vi "ValidateScanInput.vi"(0 "Original Scan":refnum<class "Scan.lvclass">, 1 "New Scan":refnum<class "Scan.lvclass">, 2 "Galvo Array":refnum<class "Galvonometer.lvclass">[](array[class])=[refnum, refnum], 3 "Camera.lvclass":refnum<class "Camera.lvclass">) -> (4 "Current Scan Schematic":cluster{dbl[], dbl[]}[](graph)=[{[-5.0, 5.0, 5.0, -5.0, -5.0], [5.0, 5.0, -5.0, -5.0, 5.0]}, {[-12.5, 12.5, 12.5, -12.5, -12.5], [12.5, 12.5, -12.5, -12.5, 12.5]}], 5 "Max file size exceeded":bool, 6 "Output scan":refnum<class "Scan.lvclass">, 7 "Memory (GB)":dbl=0.36864, 8 "Time (s)":sgl=0.72, 9 "Max Voltage Exceeded":bool)   [LabVIEW 2017]
uses:
  classes/Scans/Scan.lvclass
  classes/HardwareObjects/Galvonometer/Galvonometer.lvclass
  classes/HardwareObjects/Camera/Camera.lvclass
  classes/HardwareObjects/Camera/Camera.lvclass/Camera.ctl
  classes/HardwareObjects/Galvonometer/Galvonometer.lvclass/Galvonometer.ctl
  classes/Scans/Scan.lvclass/Scan.ctl
  classes/Scans/Write Scan Pattern.vi
  classes/Scans/Write C scans.vi
  classes/Scans/Write B scans.vi
  classes/Scans/Write Repeat B scans.vi
  classes/Scans/Write Bidirectional.vi
  classes/Scans/Write A scans.vi
  classes/Scans/Write Scan Angle (degrees).vi
  classes/Scans/Write X FOV (degrees).vi
  classes/Scans/Write X offset (degrees).vi
  classes/Scans/Write Y FOV (degrees).vi
  classes/Scans/Write Y offset (degrees).vi
  classes/HardwareObjects/Camera/Read Bit Depth.vi
  classes/HardwareObjects/Camera/Read Camera Dimensions.vi
  classes/HardwareObjects/Camera/Read Max Frequency (kHz).vi
  classes/HardwareObjects/Galvonometer/Read Max Scan Angle (degrees).vi
  classes/HardwareObjects/Galvonometer/Read Output Scale Factor (V_degrees).vi
  classes/Scans/Read Scan Pattern.vi
  classes/Scans/Read B scans.vi
  classes/Scans/Read A scans.vi
  classes/Scans/Read Scan Angle (degrees).vi
  classes/Scans/Read X FOV (degrees).vi
  classes/Scans/Read X offset (degrees).vi
  classes/Scans/Read Y FOV (degrees).vi
  classes/Scans/Read Y offset (degrees).vi
  classes/Scans/Read Total A-scans per volume.vi
panel:
  in  "stop":bool
  in  "debug":bool
  in  "Y offset (degrees)":dbl
  in  "Y FOV (degrees)":dbl=10.0
  in  "X offset (degrees)":dbl
  in  "X FOV (degrees)":dbl=10.0
  in  "Scan Angle (degrees)":dbl
  in  "A scans":dbl=300.0
  in  "Bidirectional":bool
  in  "Repeat B scans":dbl=1.0
  in  "B scans":dbl=300.0
  in  "C scans":dbl=1.0
  in  "Scan Pattern":string="Rectangle"
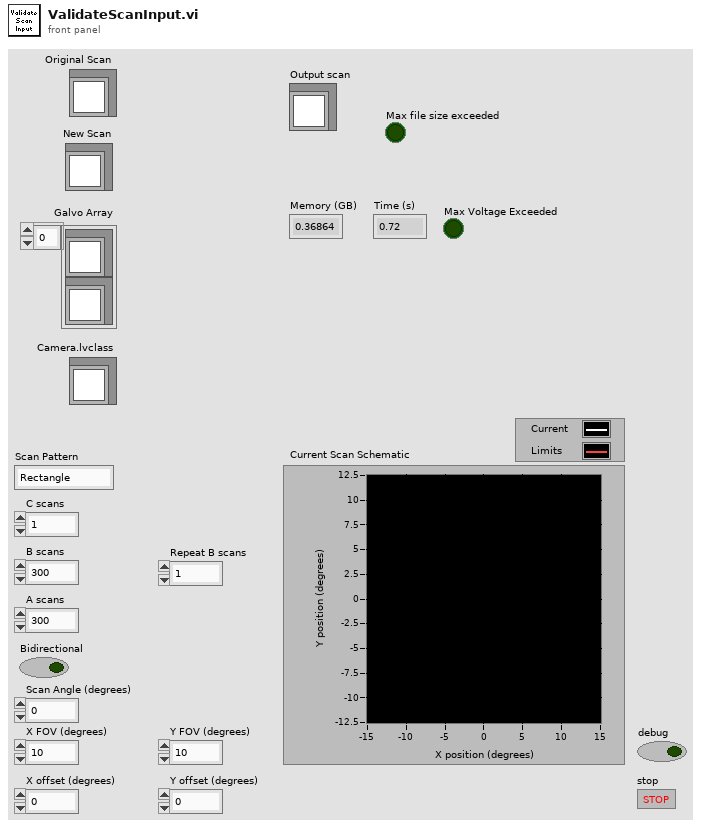
[diagram p1: front panel]
types:
  T1 = cluster{"X FOV (degrees)":dbl, "X offset (degrees)":dbl, "Y FOV (degrees)":dbl, "Y offset (degrees)":dbl}
  T2 = cluster{"X FOV (degrees)":dbl, "Y FOV (degrees)":dbl}
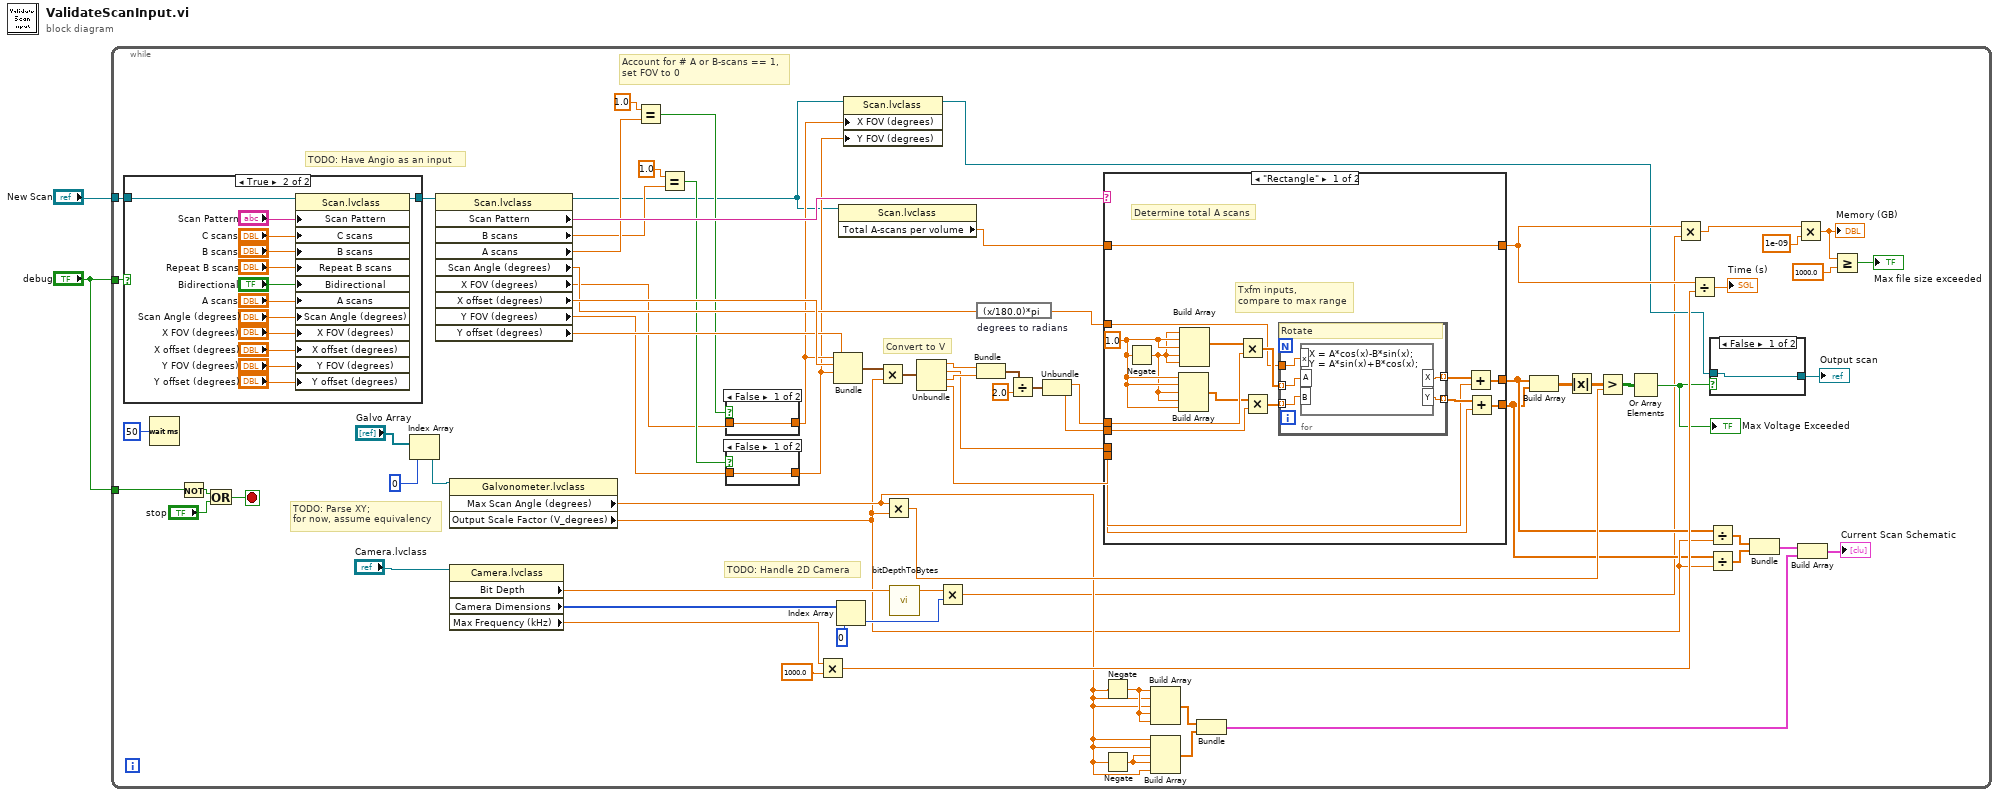
[diagram p0: block diagram]
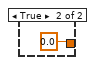
[diagram p2: hidden frame]
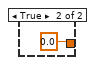
[diagram p3: hidden frame]
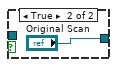
[diagram p5: hidden frame]
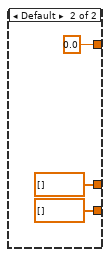
[diagram p6: hidden frame]
diagram:
  n1 = while {
    tunnel: "New Scan" -> [w33]
    tunnel: "debug" -> [w31]
    tunnel: "debug" -> [w29]
    stop <- w27 stop-if-true
    # "Account for # A or B-scans == 1,\nset FOV to 0"
    # "TODO: Have Angio as an input"
    # "TODO: Handle 2D Camera"
    # "Convert to V"
    # "TODO: Parse XY;\nfor now, assume equivalency"
    n2 = case shown="True" w31 {
      tunnel: w33 -> [w83 w85]
      tunnel: [w83 w84] -> w32
      frame False {
      }
      frame True {
        n3 = property class="Scan.lvclass"(reference=w85, "Scan Pattern"="Scan Pattern", "C scans"="C scans", "B scans"="B scans", "Repeat B scans"="Repeat B scans", "Bidirectional"="Bidirectional", "A scans"="A scans", "Scan Angle (degrees)"="Scan Angle (degrees)", "X FOV (degrees)"="X FOV (degrees)", "X offset (degrees)"="X offset (degrees)", "Y FOV (degrees)"="Y FOV (degrees)", "Y offset (degrees)"="Y offset (degrees)") -> (reference out=w84:refnum<class "Scan.lvclass">)  [unwired: 1 in, 1 out]
      }
    }
    n4 = Wait (ms)(milliseconds to wait=u32 50) -> ()  [unwired: 1 out]
    n5 = Not(x=w29) -> (.not. x?=w30:bool)
    n6 = Or(x=w30, y="stop") -> (x .or. y?=w27:bool)
    n7 = Index Array(array="Galvo Array", index=0) -> (element=w76:refnum<class "Galvonometer.lvclass">)
    n8 = property class="Scan.lvclass"(reference=w32) -> (reference out=w5:refnum<class "Scan.lvclass">, "Scan Pattern"=w74:string, "B scans"=w18:dbl, "A scans"=w20:dbl, "Scan Angle (degrees)"=w58:dbl, "X FOV (degrees)"=w15:dbl, "X offset (degrees)"=w73:dbl, "Y FOV (degrees)"=w14:dbl, "Y offset (degrees)"=w72:dbl)  [unwired: 1 in, 1 out]
    n9 = property class="Galvonometer.lvclass"(reference=w76) -> ("Max Scan Angle (degrees)"=w40:dbl, "Output Scale Factor (V_degrees)"=w39:dbl)  [unwired: 1 in, 2 out]
    n10 = property class="Camera.lvclass"(reference="Camera.lvclass") -> ("Bit Depth"=w68:dbl, "Camera Dimensions"=w70:u16[], "Max Frequency (kHz)"=w48:sgl)  [unwired: 1 in, 2 out]
    n11 = Equal?(x=1.0, y=w20) -> (x = y?=w17:bool)
    n12 = Equal?(x=1.0, y=w18) -> (x = y?=w16:bool)
    n13 = case shown="False" w17 {
      tunnel: w15 -> [w81 _]
      tunnel: [w81 0.0 ("X FOV (degrees)")] -> w13
      frame False {
      }
      frame True {
      }
    }
    n14 = case shown="False" w16 {
      tunnel: w14 -> [w79 _]
      tunnel: [w79 0.0 ("Y FOV (degrees)")] -> w12
      frame False {
      }
      frame True {
      }
    }
    n15 = Multiply(x=w48, y=1000.0) -> (x*y=w47:dbl)
    n16 = Bundle("X FOV (degrees)"=w13, "X offset (degrees)"=w73, "Y FOV (degrees)"=w12, "Y offset (degrees)"=w72) -> (w71:T1)  [unwired: 1 in]
    n17 = Index Array(array=w70, index=0) -> (element=w67:u16)
    n18 = property class="Scan.lvclass"(reference=w5) -> ("Total A-scans per volume"=w4:dbl)  [unwired: 1 in, 2 out]
    n19 = property class="Scan.lvclass"(reference=w5, "X FOV (degrees)"=w13, "Y FOV (degrees)"=w12) -> (reference out=w11:refnum<class "Scan.lvclass">)  [unwired: 1 in, 1 out]
    n20 = Multiply(x=w71, y=w39) -> (x*y=w66:T1)
    n21 = Multiply(x=w40, y=w39) -> (x*y=w53:dbl)
    n22 = call "bitDepthToBytes.vi"("bit depth"=w68) -> ("bytes"=w10:dbl)  [unwired: 9 in]
    n23 = Unbundle(w66) -> ("X FOV (degrees)"=w63:dbl, "X offset (degrees)"=w56:dbl, "Y FOV (degrees)"=w62:dbl, "Y offset (degrees)"=w55:dbl)
    n24 = Multiply(x=w10, y=w67) -> (x*y=w3:dbl)
    n25 = Bundle("X FOV (degrees)"=w63, "Y FOV (degrees)"=w62) -> (w64:T2)  [unwired: 1 in]
    n26 = expression code="(x/180.0)*pi" "degrees to radians"(w58) -> (w57:dbl)
    n27 = Divide(x=w64, y=2.0) -> (x/y=w61:T2)
    n28 = Unbundle(w61) -> ("X FOV (degrees)"=w60:dbl, "Y FOV (degrees)"=w59:dbl)
    n29 = Negate(x=w40) -> (-x=w41:dbl)
    n30 = Negate(x=w40) -> (-x=w43:dbl)
    n31 = case shown="\"Rectangle\"" w74 {
      tunnel: w60 -> [w113 _]
      tunnel: w59 -> [w112 _]
      tunnel: w57 -> [w109 _]
      tunnel: w56 -> [w106 _]
      tunnel: w55 -> [w105 _]
      tunnel: [w104 dbl[] []] -> w24
      tunnel: [w99 0.0] -> w46
      tunnel: [w103 dbl[] []] -> w23
      tunnel: w4 -> [w99 _]
      frame "Rectangle" {
        w102 = 1.0 ("element")
        # "Txfm inputs,\ncompare to max range"
        # "Determine total A scans"
        n32 = Negate(x=w102) -> (-x=w101:dbl)
        n33 = Build Array(w102, w102, w101, w101, w102) -> (w100:dbl[])
        n34 = Build Array(w101, w102, w102, w101, w101) -> (w114:dbl[])
        n35 = Multiply(x=w114, y=w113) -> (x*y=w111:dbl[])
        n36 = Multiply(x=w100, y=w112) -> (x*y=w110:dbl[])
        n37 = for {
          tunnel: w111 -> [w119] mode=indexing
          tunnel: w109 -> [w118]
          tunnel: [w117] -> w108 mode=indexing
          tunnel: w110 -> [w116] mode=indexing
          tunnel: [w115] -> w107 mode=indexing
          # "Rotate"
          n38 = formula code="X = A*cos(x)-B*sin(x);\nY = A*sin(x)+B*cos(x);"("x"=w118, "A"=w119, "B"=w116) -> ("X"=w117:dbl, "Y"=w115:dbl)
        }
        n39 = Add(x=w108, y=w106) -> (x+y=w104:dbl[])
        n40 = Add(x=w107, y=w105) -> (x+y=w103:dbl[])
      }
      frame Default {
      }
    }
    n41 = Build Array(w41, w40, w40, w41, w41) -> (w44:dbl[])
    n42 = Build Array(w40, w40, w43, w43, w40) -> (w42:dbl[])
    n43 = Bundle(w44, w42) -> (w35:cluster{dbl[], dbl[]})  [unwired: 1 in]
    n44 = Build Array(w24, w23) -> (w22:dbl[][])
    n45 = Absolute Value(x=w22) -> (abs(x)=w54:dbl[][])
    n46 = Greater?(x=w54, y=w53) -> (0:w51:bool[][])
    n47 = Or Array Elements(Boolean array=w51) -> (logical OR=w25:bool)
    "Max Voltage Exceeded" <- w25
    n48 = Multiply(x=w46, y=w3) -> (x*y=w7:dbl)
    n49 = Divide(x=w46, y=w47) -> (x/y=→"Time (s)":dbl)
    n50 = Divide(x=w24, y=w39) -> (x/y=w38:dbl[])
    n51 = Divide(x=w23, y=w39) -> (x/y=w37:dbl[])
    n52 = case shown="False" w25 {
      tunnel: [w97 "Original Scan"] -> w50
      tunnel: w11 -> [w97 _]
      frame False {
      }
      frame True {
      }
    }
    "Output scan" <- w50
    n53 = Bundle(w38, w37) -> (w36:cluster{dbl[], dbl[]})  [unwired: 1 in]
    n54 = Multiply(x=w7, y=1e-09) -> (x*y=w6:dbl)
    "Memory (GB)" <- w6
    n55 = Build Array(w36, w35) -> (→"Current Scan Schematic":cluster{dbl[], dbl[]}[])
    n56 = Greater Or Equal?(x=w6, y=1000.0) -> (x >= y?=→"Max file size exceeded":bool)
  }
